vi "For循环的使用(上).vi"() -> ()   [LabVIEW 2018]
panel:
  out "提示":bool
  out "当前循环次数":dbl
  in  "数值输入":dbl
  out "显示":dbl
  in  "输入":dbl
  out "数值":i32
  # "计算4+9+16+...+x^2。(x为输入的值)"
  # "程序循环产生1000次小于1000的随机数，若本次产生的数与输入的数一致，则打印当前循环次数。若都不一致则进行提示。"
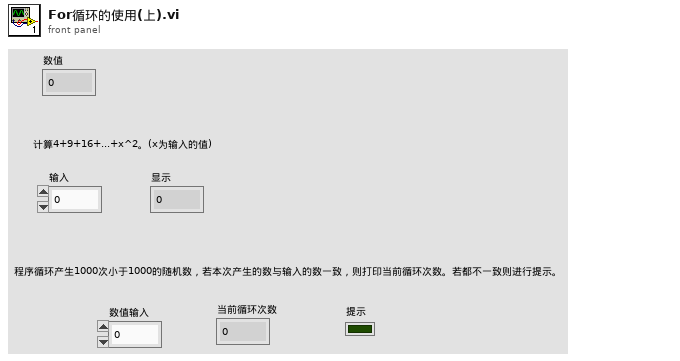
[diagram p1: front panel]
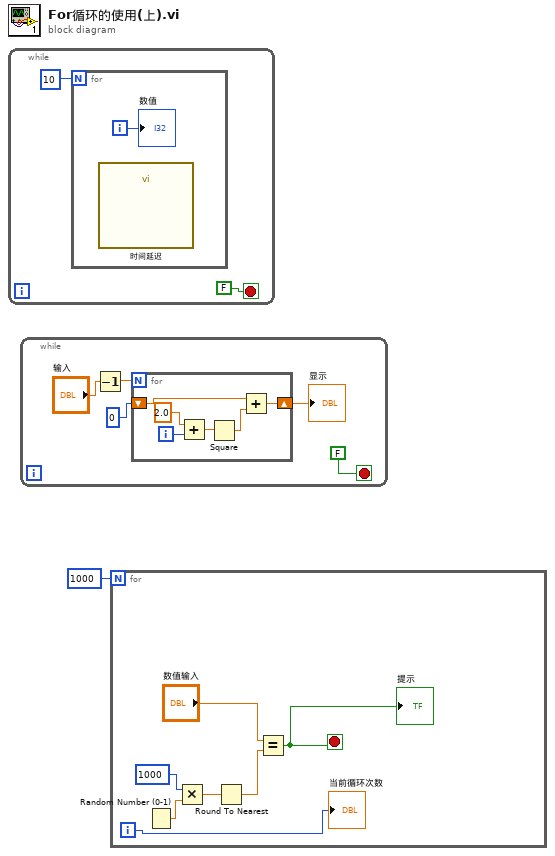
[diagram p0: block diagram]
diagram:
  n1 = while {
    stop <- FALSE stop-if-true
    n2 = for {
      N: 10 -> [_]
      i -> [w4]
      n3 = call "时间延迟"() -> ()  [unwired: 11 in, 1 out]
      "数值" <- w4
    }
  }
  n4 = while {
    stop <- FALSE stop-if-true
    n5 = Decrement(x="输入") -> (x-1=w7:dbl)
    n6 = for {
      N: w7 -> [_]
      shift-right: [w10] -> w5
      shift-left: 0 -> [w12]
      i -> [w14]
      n7 = Add(x=2.0, y=w14) -> (x+y=w13:dbl)
      n8 = Square(x=w13) -> (x^2=w11:dbl)
      n9 = Add(x=w12, y=w11) -> (x+y=w10:dbl)
    }
    "显示" <- w5
  }
  n10 = for {
    N: 1000 -> [_]
    i -> [w17]
    stop <- w16 stop-if-true
    n11 = Random Number (0-1)() -> (number: 0 to 1=w21:dbl)
    n12 = Multiply(x=1000, y=w21) -> (x*y=w20:dbl)
    n13 = Round To Nearest(number=w20) -> (nearest integer value=w19:dbl)
    n14 = Equal?(x="数值输入", y=w19) -> (x = y?=w16:bool)
    "提示" <- w16
    "当前循环次数" <- w17
  }
